vi "lab2_Shimeng_LI.vi"(0 "String Input":string) -> (1 "x local":dbl, 2 "y local":dbl)   [LabVIEW 2014]
panel:
  out "horizontal distance":dbl
  out "Slope Distance number":dbl
  out "V number":dbl
  out "Hz number":dbl
  out "Slope Distance":string
  out "V":string
  out "Hz":string
  out "before substring":string
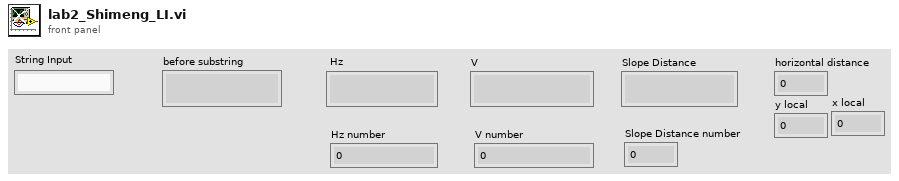
[diagram p1: front panel]
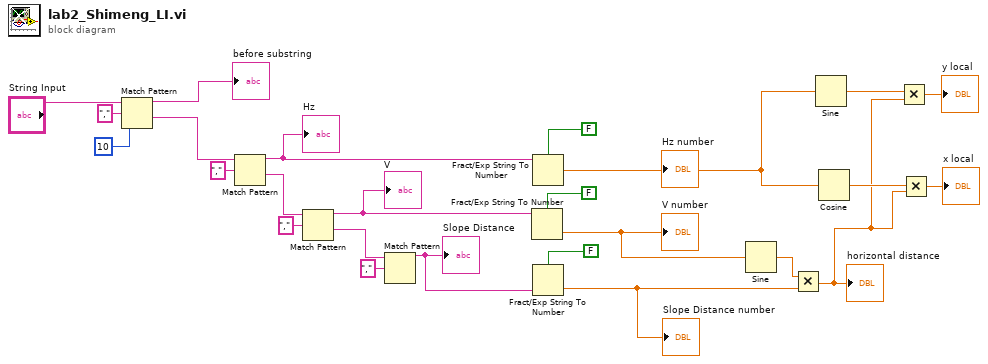
[diagram p0: block diagram]
diagram:
  n1 = Match Pattern(string="String Input", regular expression=",", offset (0)=10) -> (before substring=→"before substring":string, after substring=w21:string)  [unwired: 2 out]
  n2 = Match Pattern(string=w21, regular expression=",") -> (before substring=w15:string, after substring=w19:string)  [unwired: 1 in, 2 out]
  "Hz" <- w15
  n3 = Match Pattern(string=w19, regular expression=",") -> (before substring=w14:string, after substring=w17:string)  [unwired: 1 in, 2 out]
  "V" <- w14
  n4 = Match Pattern(string=w17, regular expression=",") -> (before substring=w13:string)  [unwired: 1 in, 3 out]
  "Slope Distance" <- w13
  n5 = Fract/Exp String To Number(use system decimal point (T)=FALSE, string=w14) -> (number=w8:dbl)  [unwired: 2 in, 1 out]
  "V number" <- w8
  n6 = Fract/Exp String To Number(use system decimal point (T)=FALSE, string=w15) -> (number=w6:dbl)  [unwired: 2 in, 1 out]
  "Hz number" <- w6
  n7 = Fract/Exp String To Number(use system decimal point (T)=FALSE, string=w13) -> (number=w7:dbl)  [unwired: 2 in, 1 out]
  "Slope Distance number" <- w7
  n8 = Sine(x=w8) -> (sin(x)=w9:dbl)
  n9 = Multiply(x=w9, y=w7) -> (x*y=w3:dbl)
  "horizontal distance" <- w3
  n10 = Sine(x=w6) -> (sin(x)=w5:dbl)
  n11 = Cosine(x=w6) -> (cos(x)=w4:dbl)
  n12 = Multiply(x=w5, y=w3) -> (x*y=→"y local":dbl)
  n13 = Multiply(x=w4, y=w3) -> (x*y=→"x local":dbl)
